vi "dsdll_generate_error.vi"(6 "error code":i32, 8 "error in":errorcluster, 9 "dsdll instance in":T1) -> (0 "error out":errorcluster, 1 "dsdll instance out":T1, 4 "error string":string)   [LabVIEW 2018, in "dsdll.lvlib"]
doc: "Call this to convert DSDLL error code to string and generate error into error wire."
uses:
  dsdll.lvlib
  dsdll_instance.ctl
  dsdll_device_record.ctl
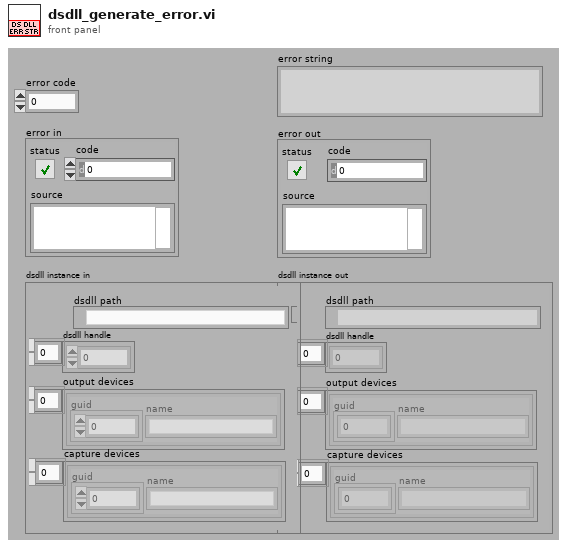
[diagram p1: front panel]
types:
  T1 = typedef "dsdll.lvlib/dsdll_instance.ctl" = cluster{"dsdll path":path, "dsdll handle":u8[], "output devices":T2[], "capture devices":T2[]}
  T2 = typedef "dsdll.lvlib/dsdll_device_record.ctl" = cluster{"guid":u8[], "name":string}
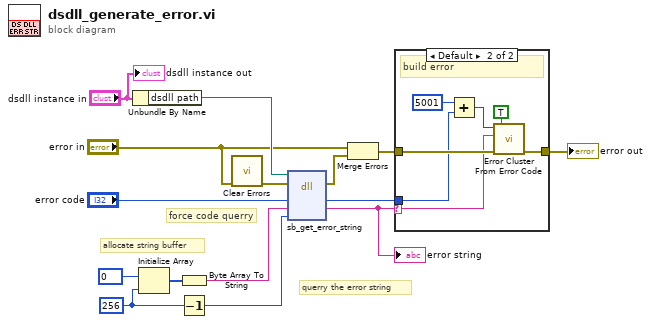
[diagram p0: block diagram]
diagram:
  w15 = 256 ("strlen")
  # "querry the error string"
  # "force code querry"
  # "allocate string buffer"
  n1 = Unbundle By Name("dsdll instance in") -> ("dsdll path"=w10:path)
  n2 = Initialize Array(u8 0, w15) -> (w13:u8[])
  n3 = Byte Array To String(unsigned byte array=w13) -> (string=w12:string)
  n4 = Decrement(x=w15) -> (x-1=w7:i32)
  n5 = call <vilib>:"Clear Errors.vi"("error in (no error)"="error in") -> ("error out"=w6:errorcluster)  [unwired: 5 in, 1 out]
  n6 = dll-call lib="dsdll.dll" fn="sb_get_error_string" ("sb_get_handle_size()")(path in=w10, error in=w6, "code"="error code", "str"=w12, "strlen"=w7) -> (error out=w8:errorcluster, "code"=w3:i32, "str"=w2:string)  [unwired: 3 in, 1 out]
  "error string" <- w2
  n7 = Merge Errors("error in", w8) -> (w4:errorcluster)
  n8 = case shown="Default" w2 {
    selector: w2 -> [_ w18]
    tunnel: w4 -> [w16 w23]
    tunnel: w3 -> [_ w20]
    tunnel: [w16 w17] -> w1
    frame "" {
    }
    frame Default {
      # "build error"
      n9 = Add(x=5001, y=w20) -> (x+y=w19:i32)
      n10 = call <vilib>:"Error Cluster From Error Code.vi"("show call chain? (False)"=TRUE, "error in (no error)"=w23, "error message (\"\")"=w18, "error code (0)"=w19) -> ("error out"=w17:errorcluster)  [unwired: 5 in]
    }
  }
  "error out" <- w1
  "dsdll instance out" <- "dsdll instance in"
